vi "Write Sync Group.vi"(8 "error in (no error)":errorcluster, 10 "Sync Group":u8=128 format="%x", 11 "DriveMotorsRight in":refnum<class "DriveMotorsRight.lvclass">) -> (0 "error out":errorcluster, 3 "DriveMotorsRight out":refnum<class "DriveMotorsRight.lvclass">)   [LabVIEW 2013, in "DriveMotorsRight.lvclass"]
uses:
  DriveMotorsRight.lvclass
  DriveMotorsRight.lvclass/DriveMotorsRight.ctl
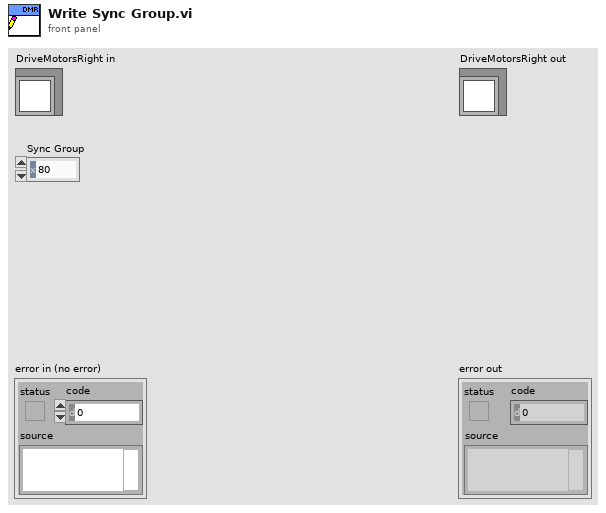
[diagram p1: front panel]
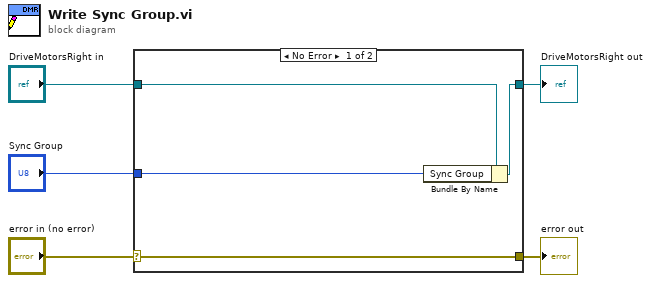
[diagram p0: block diagram]
diagram:
  n1 = case shown="No Error" "error in (no error)" {
    selector: "error in (no error)" -> [w9 w10]
    tunnel: [w9 w10] -> w4
    tunnel: [w7 w11] -> w2
    tunnel: "DriveMotorsRight in" -> [w8 w11]
    tunnel: "Sync Group" -> [w6 _]
    frame No Error {
      n2 = Bundle By Name(cluster=w8, "Sync Group"=w6) -> (w7:refnum<class "DriveMotorsRight.lvclass">)
    }
    frame Error {
    }
  }
  "error out" <- w4
  "DriveMotorsRight out" <- w2
